vi "采集数据保存sql.vi"(9 "标识":string, 10 "表名":string, 11 "簇":T2 {"反应温度" format="%.1f"}) -> ()   [LabVIEW 2023]
panel:
  out "连接的字符串":string
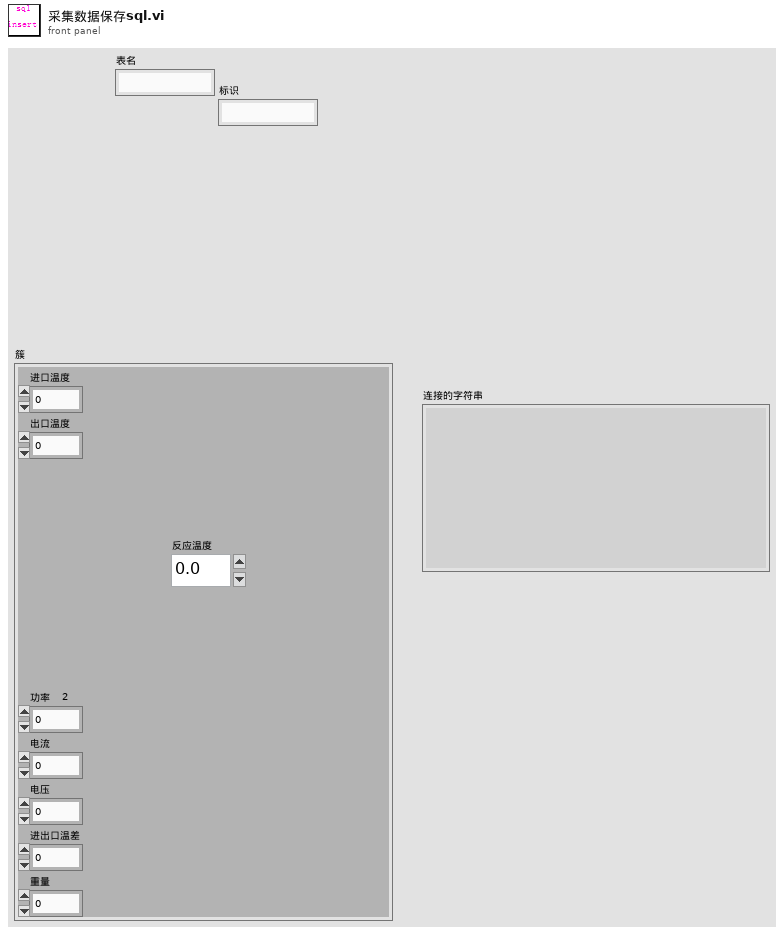
[diagram p1: front panel]
types:
  T1 = typedef "控件 13.ctl" = dbl
  T2 = cluster{"进口温度":dbl, "出口温度":dbl, "反应温度":T1, "功率    2":dbl, "电流":dbl, "电压":dbl, "进出口温差":dbl, "重量":dbl}
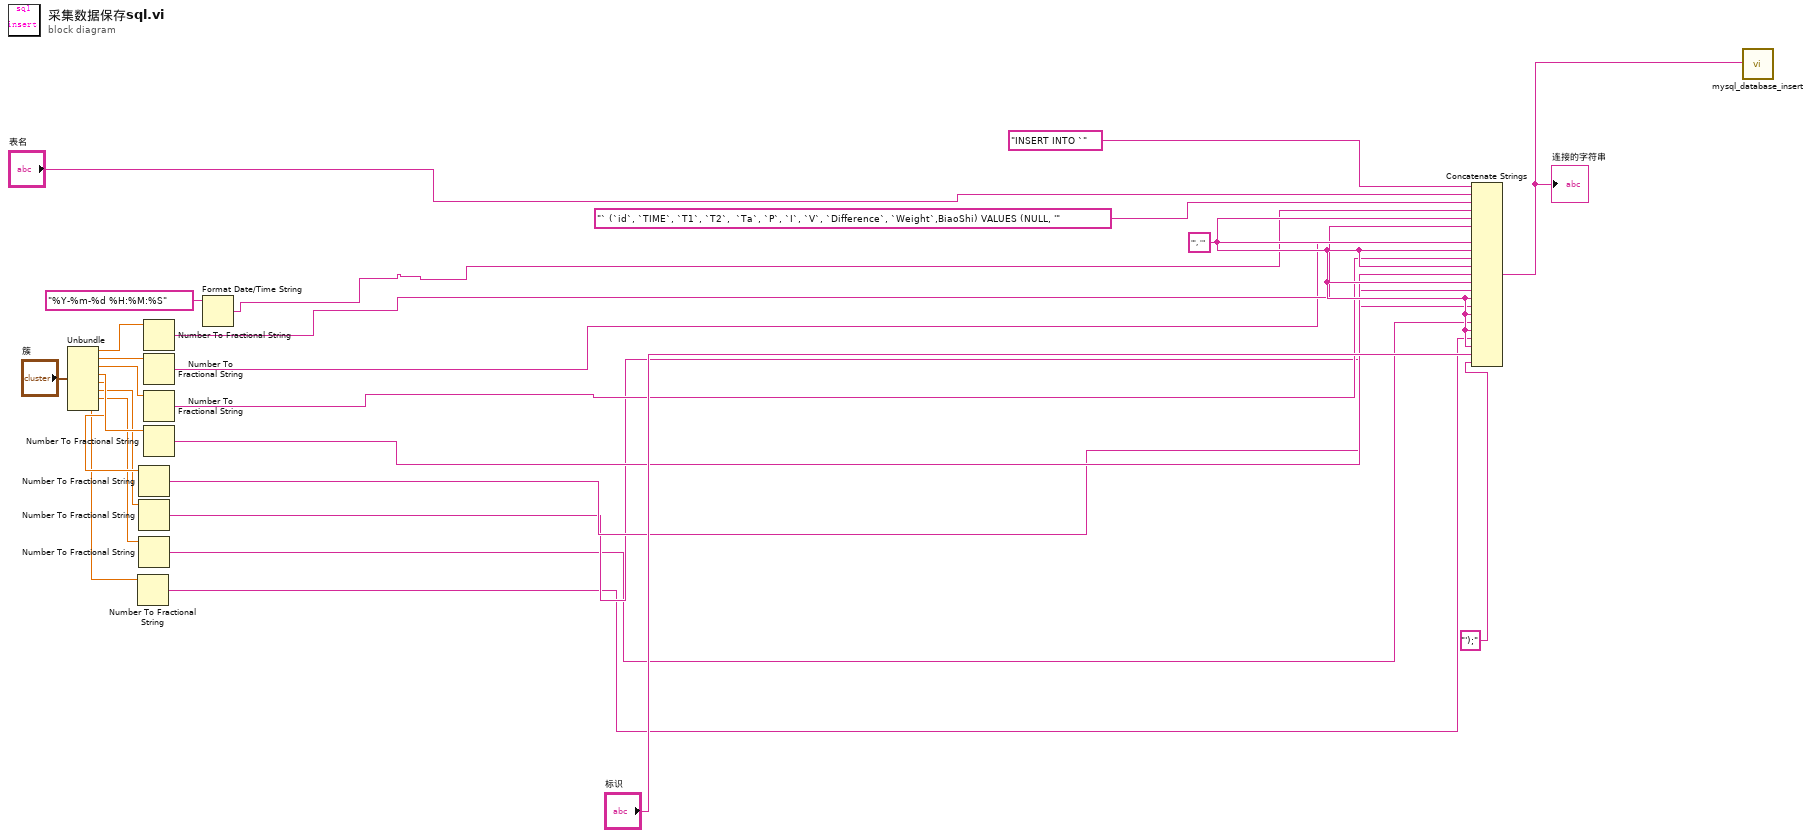
[diagram p0: block diagram]
diagram:
  w23 = "', '" ("字符串")
  n1 = Unbundle("簇") -> ("进口温度"=w20:dbl, "出口温度"=w19:dbl, "反应温度"=w17:T1, "功率    2"=w16:dbl, "电流"=w15:dbl, "电压"=w14:dbl, "进出口温差"=w13:dbl, "重量"=w12:dbl)
  n2 = Number To Fractional String(number=w12) -> (F-format string=w1:string)  [unwired: 3 in]
  n3 = Number To Fractional String(number=w15) -> (F-format string=w4:string)  [unwired: 3 in]
  n4 = Number To Fractional String(number=w14) -> (F-format string=w3:string)  [unwired: 3 in]
  n5 = Number To Fractional String(number=w13) -> (F-format string=w2:string)  [unwired: 3 in]
  n6 = Number To Fractional String(number=w20) -> (F-format string=w8:string)  [unwired: 3 in]
  n7 = Number To Fractional String(number=w19) -> (F-format string=w7:string)  [unwired: 3 in]
  n8 = Number To Fractional String(number=w17) -> (F-format string=w6:string)  [unwired: 3 in]
  n9 = Number To Fractional String(number=w16) -> (F-format string=w5:string)  [unwired: 3 in]
  n10 = Format Date/Time String(time format string (%c)="%Y-%m-%d %H:%M:%S" ("时间格式字符串(%c)")) -> (date/time string=w9:string)  [unwired: 2 in]
  n11 = Concatenate Strings("INSERT INTO `" ("字符串"), "表名", "` (`id`, `TIME`, `T1`, `T2`,  `Ta`, `P`, `I`, `V`, `Difference`, `Weight`,BiaoShi) VALUES (NULL, '" ("字符串"), w9, w23, w8, w23, w7, w23, w6, w23, w5, w23, w4, w23, w3, w23, w2, w23, w1, w23, "标识", "');" ("字符串")) -> (w21:string)
  "连接的字符串" <- w21
  n12 = call "mysql_database_insert.vi"("SQL query"=w21) -> ()  [unwired: 1 in]
